vi "Panel Initialize.vi"(8 "error in":errorcluster, 10 "Initialize All UI ?":bool, 11 "VI Ref":refnum<vi>) -> (0 "error out":errorcluster, 1 "Ver.#":string, 3 "Structure Data":T1)   [LabVIEW 2020]
uses:
  Def/Main_Data_Package.ctl
  Def/User_Event.ctl
  Def/Initialize table.ctl
  Def/Queue_Method Def.ctl
  <vilib>/Utility/Data Type/NI_Data Type.lvlib
panel:
  in  "Structure Data":T1
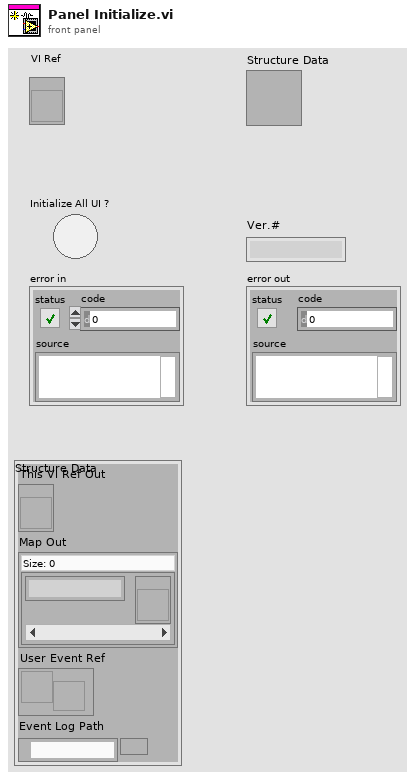
[diagram p1: front panel]
types:
  T1 = typedef "Main_Data_Package.ctl" = cluster{"This Vi Ref Out":refnum<vi>, "Map Out":map{string, refnum<vi>}, "User Event Ref":refnum<user-event>, "Event Log Path":path}
  T2 = typedef "Initialize table.ctl" = enum16{"Get Main Panel UI Ref", "User event Initialize", "Arc Queue Initialize", "Arc Notifier Initialize", "Load Event Log  Path", "Other procedure"}
  T3 = enum16{"Initialize", "Get", "Read", "Write", "Release"}
  T4 = enum16{"Initialize", "Write", "Read", "Release All Notifiers"}
  T5 = typedef "Queue_Method Def.ctl" = enum16{"Initialize", "Read", "Write", "Insert", "Get_Specific_Quene_Status", "Flush Speciffic Quene", "Release All Quenes"}
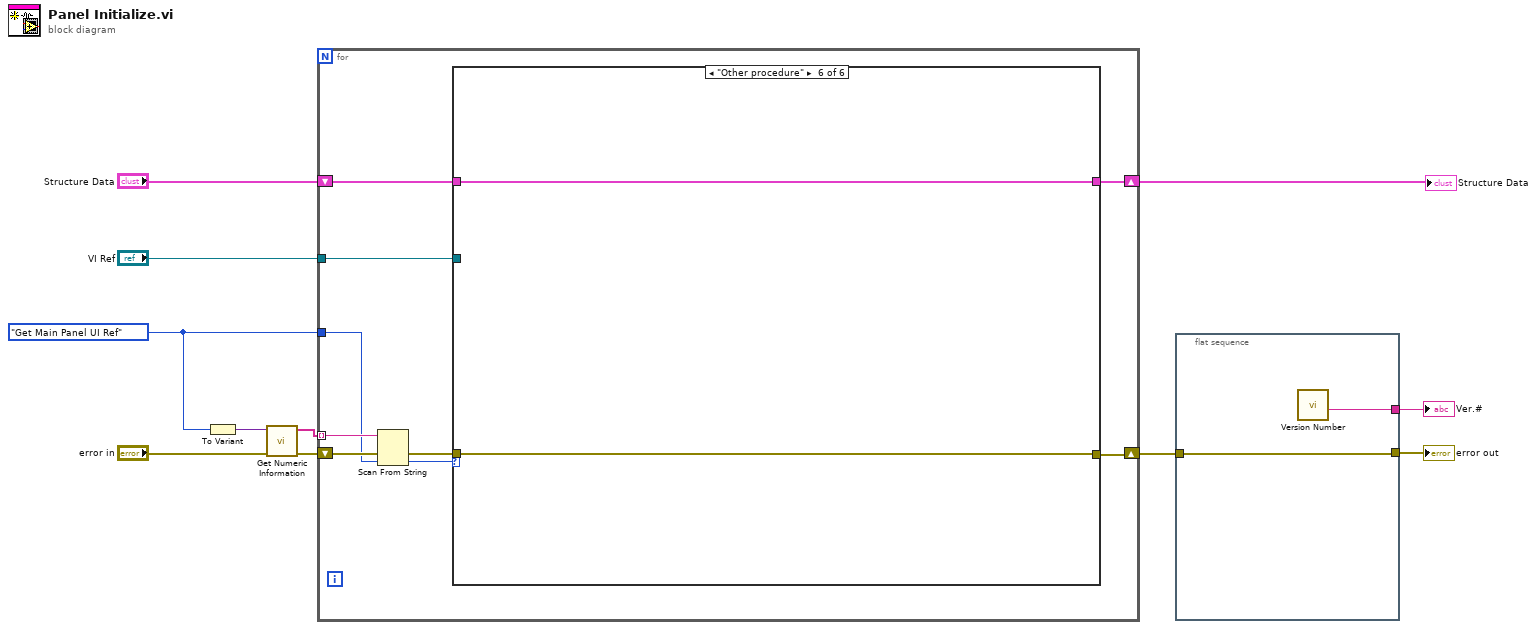
[diagram p0: block diagram]
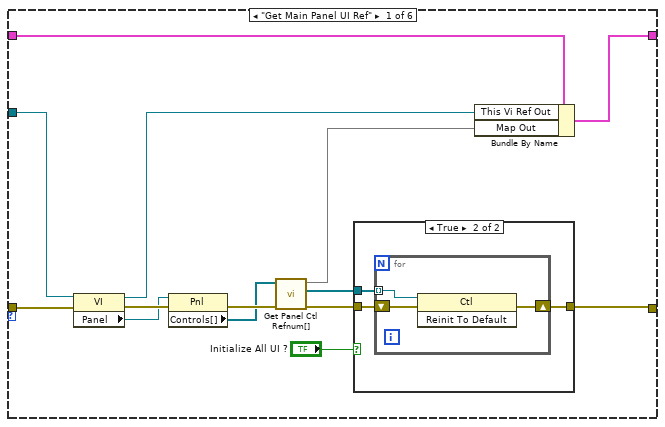
[diagram p2: hidden frame]
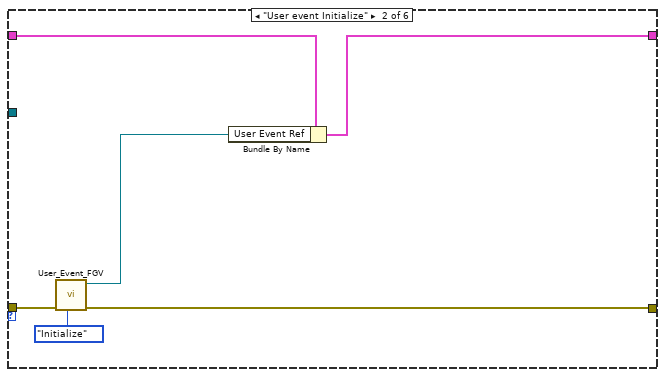
[diagram p4: hidden frame]
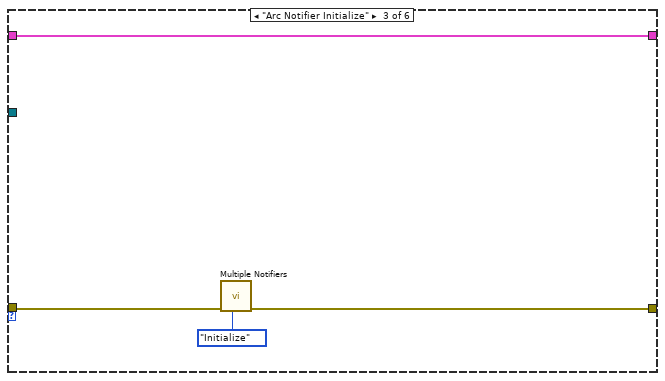
[diagram p5: hidden frame]
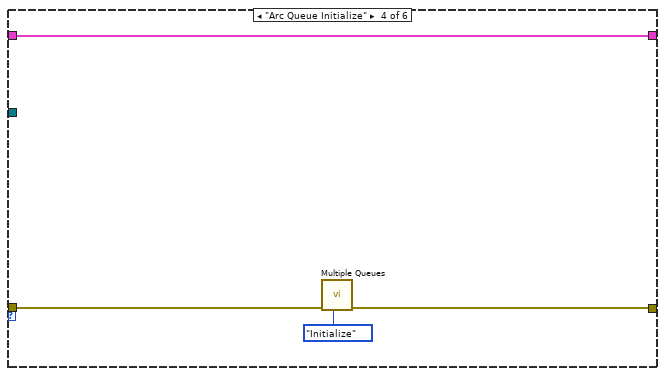
[diagram p6: hidden frame]
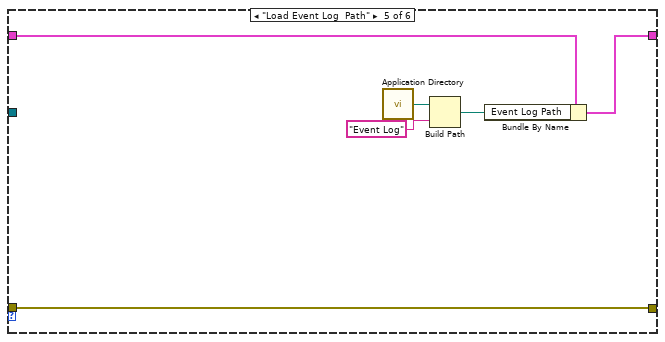
[diagram p7: hidden frame]
diagram:
  w3 = Initialize_table."Get Main Panel UI Ref"
  n1 = To Variant(anything=w3) -> (Variant=w5:variant)
  n2 = call <vilib>:"Get Numeric Information.vi"("error in (no error)"="error in", "variant"=w5) -> ("error out"=w6:errorcluster, "enum names"=w4:string[])  [unwired: 6 in, 2 out]
  n3 = for {
    shift-right: [w14] -> w8
    shift-left: w6 -> [w18]
    tunnel: w4 -> [w19] mode=indexing
    tunnel: w3 -> [w17]
    tunnel: "VI Ref" -> [w20]
    shift-right: [w12] -> w1
    shift-left: "Structure Data" -> [w13]
    n4 = Scan From String(input string=w19, error in=w18, default 1=w17) -> (error out=w15:errorcluster, output 1=w16:T2)  [unwired: 2 in, 2 out]
    n5 = case shown="\"Other procedure\"" w16 {
      tunnel: w20 -> [w34 _ _ _ _ _]
      tunnel: w15 -> [w33 w46 w48 w53 w61 w63]
      tunnel: [w32 w45 w49 w52 w61 w63] -> w14
      tunnel: w13 -> [w31 w44 w50 w55 w58 w62]
      tunnel: [w30 w43 w50 w55 w57 w62] -> w12
      frame "Get Main Panel UI Ref" {
        n6 = property on="Property Node" class="VI"(reference=w34, error in=w33) -> (reference out=w22:refnum<vi>, error out=w29:errorcluster, "Panel"=w28:refnum<vi>)
        n7 = property on="Property Node" class="Pnl"(reference=w28, error in=w29) -> (error out=w26:errorcluster, "Controls[]"=w23:refnum<vi>[])  [unwired: 1 out]
        n8 = call "Get Panel Ctl Refnum[].vi"("error in"=w26, "Controls[]"=w23) -> ("error out"=w25:errorcluster, "Controls[] Out"=w24:refnum<vi>[], "Map Out"=w21:map{string, refnum<vi>})  [unwired: 7 in]
        n9 = case shown="True" "Initialize All UI ?" {
          tunnel: [w35 w38] -> w32
          tunnel: w25 -> [w35 w37]
          tunnel: w24 -> [_ w36]
          frame False {
          }
          frame True {
            n10 = for {
              shift-right: [w40] -> w38
              shift-left: w37 -> [w41]
              tunnel: w36 -> [w39] mode=indexing
              n11 = invoke class="Ctl" method="Reinit To Default"(reference=w39, error in=w41) -> (error out=w40:errorcluster)  [unwired: 1 in, 2 out]
            }
          }
        }
        n12 = Bundle By Name(cluster=w31, "This Vi Ref Out"=w22, "Map Out"=w21) -> (w30:T1)
      }
      frame "User event Initialize" {
        n13 = call "User_Event_FGV.vi"("Method"=T3."Initialize", "error in"=w46) -> ("error out"=w45:errorcluster, "User Event Out"=w42:refnum<user-event>)  [unwired: 8 in]
        n14 = Bundle By Name(cluster=w44, "User Event Ref"=w42) -> (w43:T1)
      }
      frame "Arc Notifier Initialize" {
        n15 = call "Multiple Notifiers.vi"("Method"=T4."Initialize", "error in (no error)"=w48) -> ("error out"=w49:errorcluster)  [unwired: 8 in, 1 out]
      }
      frame "Arc Queue Initialize" {
        n16 = call "Multiple Queues.vi"("Method"=Queue_Method_Def."Initialize", "error in"=w53) -> ("error out"=w52:errorcluster)  [unwired: 7 in, 2 out]
      }
      frame "Load Event Log  Path" {
        n17 = call <vilib>:"Application Directory.vi"() -> ("Application Directory"=w60:path)
        n18 = Build Path(base path=w60, name or relative path="Event Log") -> (appended path=w56:path)
        n19 = Bundle By Name(cluster=w58, "Event Log Path"=w56) -> (w57:T1)
      }
      frame "Other procedure" {
      }
    }
  }
  "Structure Data" <- w1
  n20 = flat-sequence {
    tunnel: [w64] -> w10
    tunnel: [w65] -> w9
    tunnel: w8 -> [w64]
    frame #0 {
      # "First Step"
      n21 = call "Version Number.vi"() -> ("Version Number"=w65:string)  [unwired: 11 in]
    }
  }
  "error out" <- w10
  "Ver.#" <- w9
